vi "3.2.vi"(8 "error in (no error)":errorcluster, 10 "String":string) -> (0 "error out":errorcluster, 2 "Numeric":i32)   [LabVIEW 2017]
panel:
  out "number 2":u32
  out "number":u32
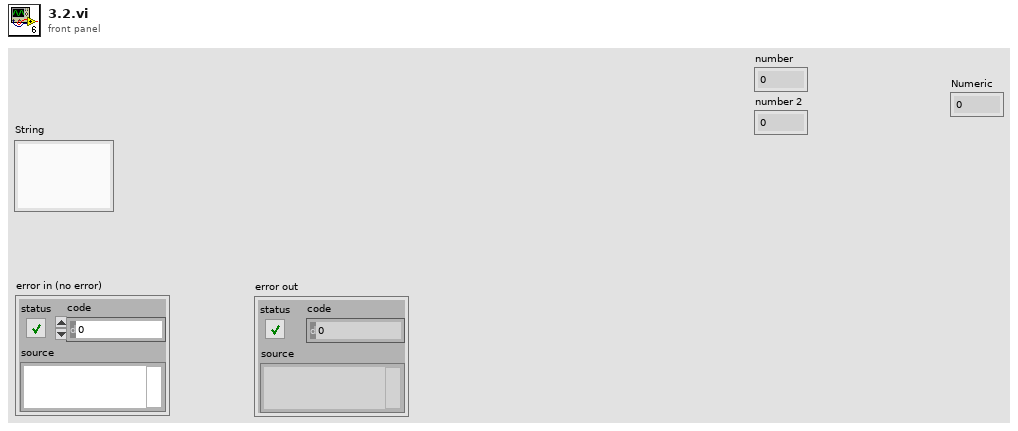
[diagram p1: front panel]
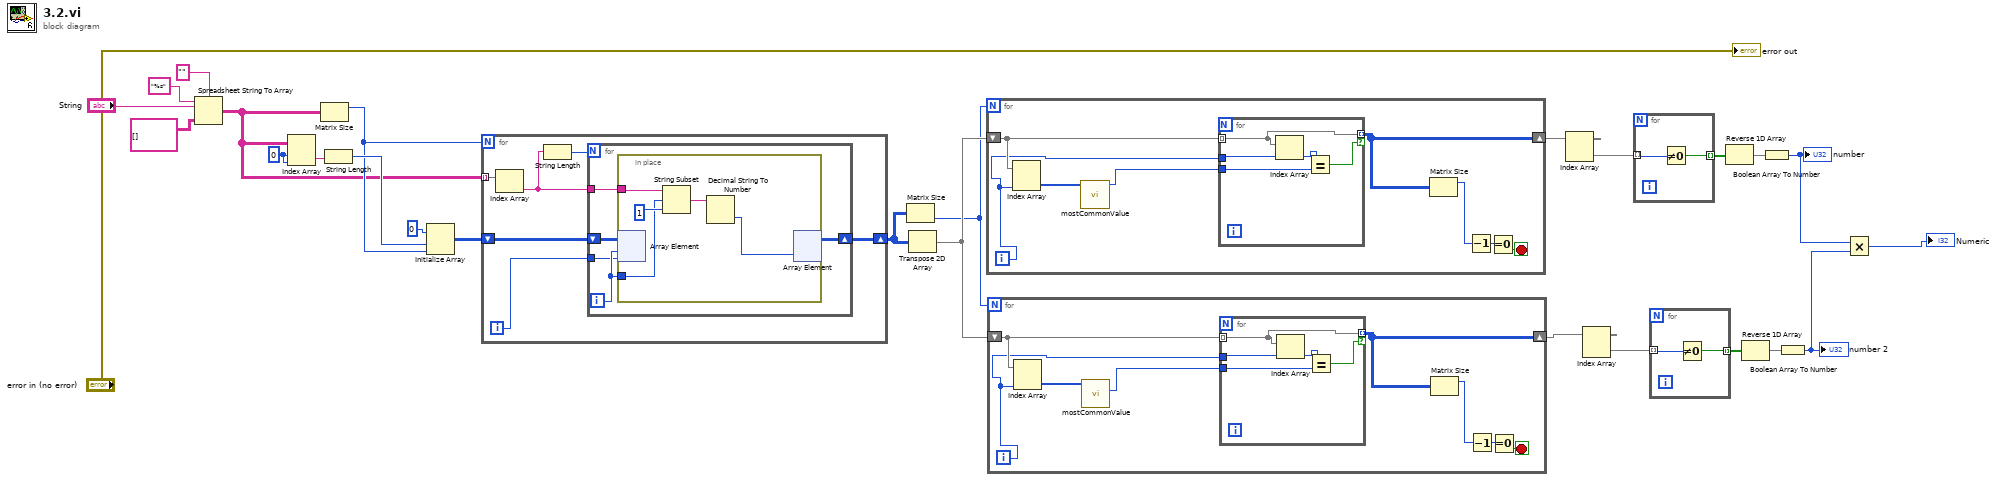
[diagram p0: block diagram]
diagram:
  w22 = 0 ("index (row)")
  n1 = Spreadsheet String To Array(delimiter (Tab)="", format string="%s", spreadsheet string="String", array type (2D Dbl)=string[][] []) -> (array=w16:string[][])
  n2 = Index Array(array=w16, index (row)=w22, index (col)=w22) -> (element=w21:string)
  n3 = Matrix Size(0:w16) -> (1:w17:i32)  [unwired: 1 out]
  n4 = String Length(string=w21) -> (length=w19:i32)
  n5 = Initialize Array(0 ("element"), w19, w17) -> (w18:i32[][])
  n6 = for {
    N: w17 -> [_]
    tunnel: w16 -> [w30] mode=indexing
    shift-right: [w27] -> w14
    shift-left: w18 -> [w32]
    i -> [w31]
    n7 = Index Array(array=w30) -> (element=w29:string)  [unwired: 1 in]
    n8 = String Length(string=w29) -> (length=w28:i32)
    n9 = for {
      N: w28 -> [_]
      shift-right: [w35] -> w27
      shift-left: w32 -> [w37]
      tunnel: w31 -> [w33]
      tunnel: w29 -> [w36]
      i -> [w34]
      n10 = in-place {
        in-place-border: w36 -> [w41]
        in-place-border: w34 -> [w40]
        n11 = in-place-array #1(w37, w34, w33) -> ()  [unwired: 1 out]
        n12 = String Subset(string=w41, offset (0)=w40, length (rest)=1 ("length (rest)")) -> (substring=w39:string)
        n13 = Decimal String To Number(string=w39) -> (number=w38:i32)  [unwired: 2 in, 1 out]
        n14 = in-place-array #1(w38) -> (w35:i32[][])  [unwired: 2 out]
      }
    }
  }
  n15 = Matrix Size(0:w14) -> (2:w8:i32)  [unwired: 1 out]
  n16 = Transpose 2D Array(2D array=w14) -> (transposed array=w9:i32[][])
  n17 = for {
    N: w8 -> [_]
    shift-right: [w47] -> w13
    shift-left: w9 -> [w48]
    i -> [w44]
    stop <- w45 stop-if-true
    n18 = Index Array(array=w48, index (col)=w44) -> (element=w50:i32[])  [unwired: 1 in]
    n19 = call "mostCommonValue.vi"("Array"=w50) -> ("Major"=w49:i32)  [unwired: 9 in, 1 out]
    n20 = for {
      tunnel: w48 -> [w52] mode=indexing
      tunnel: w44 -> [w55]
      tunnel: w49 -> [w53]
      tunnel: [w52] -> w47 mode=indexing if=w51
      n21 = Index Array(array=w52, index=w55) -> (element=w54:i32)
      n22 = Equal?(x=w54, y=w53) -> (x = y?=w51:bool)
    }
    n23 = Matrix Size(0:w47) -> (1:w43:i32)  [unwired: 1 out]
    n24 = Decrement(x=w43) -> (x-1=w46:i32)
    n25 = Equal To 0?(x=w46) -> (x = 0?=w45:bool)
  }
  n26 = for {
    N: w8 -> [_]
    shift-right: [w61] -> w4
    shift-left: w9 -> [w62]
    i -> [w58]
    stop <- w59 stop-if-true
    n27 = Index Array(array=w62, index (col)=w58) -> (element=w63:i32[])  [unwired: 1 in]
    n28 = call "mostCommonValue.vi"("Array"=w63) -> ("Minor"=w56:i32)  [unwired: 9 in, 1 out]
    n29 = for {
      tunnel: w62 -> [w65] mode=indexing
      tunnel: w58 -> [w68]
      tunnel: w56 -> [w66]
      tunnel: [w65] -> w61 mode=indexing if=w64
      n30 = Index Array(array=w65, index=w68) -> (element=w67:i32)
      n31 = Equal?(x=w67, y=w66) -> (x = y?=w64:bool)
    }
    n32 = Matrix Size(0:w61) -> (1:w57:i32)  [unwired: 1 out]
    n33 = Decrement(x=w57) -> (x-1=w60:i32)
    n34 = Equal To 0?(x=w60) -> (x = 0?=w59:bool)
  }
  n35 = Index Array(array=w13) -> (element=w12:i32[])  [unwired: 2 in]
  n36 = Index Array(array=w4) -> (element=w5:i32[])  [unwired: 2 in]
  n37 = for {
    tunnel: w12 -> [w70] mode=indexing
    tunnel: [w69] -> w11 mode=indexing
    n38 = Not Equal To 0?(x=w70) -> (x != 0?=w69:bool)
  }
  n39 = for {
    tunnel: w5 -> [w72] mode=indexing
    tunnel: [w71] -> w6 mode=indexing
    n40 = Not Equal To 0?(x=w72) -> (x != 0?=w71:bool)
  }
  n41 = Reverse 1D Array(array=w11) -> (reversed array=w10:bool[])
  n42 = Reverse 1D Array(array=w6) -> (reversed array=w7:bool[])
  n43 = Boolean Array To Number(Boolean array=w10) -> (number=w3:u32)
  "number" <- w3
  n44 = Boolean Array To Number(Boolean array=w7) -> (number=w2:u32)
  "number 2" <- w2
  n45 = Multiply(x=w3, y=w2) -> (x*y=→"Numeric":u32)
  "error out" <- "error in (no error)"
